vi "ep_Load Torque Efficiency (1 Chan).vi"(1 "additional efficiency information":T1, 7 "speed [RPM]":dbl, 11 "error in (no error)":errorcluster, 12 "nameplate information":T2, 13 "total input active power [W]":dbl) -> (4 "torque [Nm]":dbl, 6 "load [kW]":dbl, 8 "efficiency [%]":dbl, 15 "error out":errorcluster)   [LabVIEW 2014, in "NI_EP_Motor Monitoring.lvlib"]
uses:
  <vilib>/addons/Electrical Power/Motor Monitoring/NI_EP_Motor Monitoring.lvlib
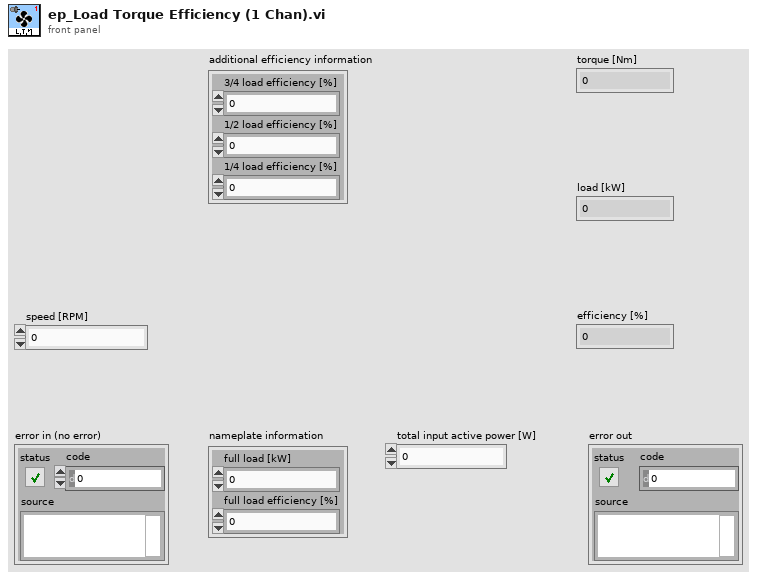
[diagram p1: front panel]
types:
  T1 = cluster{"3/4 load efficiency [%]":dbl, "1/2 load efficiency [%]":dbl, "1/4 load efficiency [%]":dbl}
  T2 = cluster{"full load [kW]":dbl, "full load efficiency [%]":dbl}
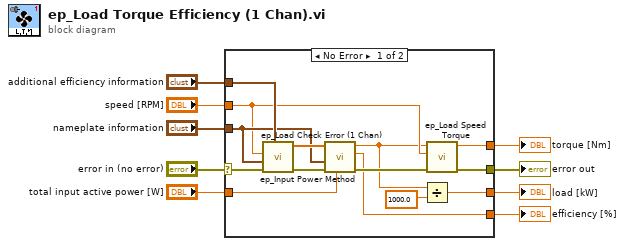
[diagram p0: block diagram]
diagram:
  n1 = case shown="No Error" "error in (no error)" {
    selector: "error in (no error)" -> [w23 w24]
    tunnel: [w15 w24] -> w8
    tunnel: "total input active power [W]" -> [w18 _]
    tunnel: "nameplate information" -> [w19 _]
    tunnel: "speed [RPM]" -> [w16 _]
    tunnel: "additional efficiency information" -> [w22 _]
    tunnel: [w14 _] -> w3
    tunnel: [w11 _] -> w2
    tunnel: [w13 _] -> w1
    frame No Error {
      n2 = call <vilib>:"ep_Load Check Error (1 Chan).vi"("additional efficiency information"=w22, "error in (no error)"=w23, "nameplate information"=w19, "speed [RPM]"=w16) -> ("error out"=w21:errorcluster, "efficiency values [%]"=w20:dbl[])  [unwired: 6 in]
      n3 = call <vilib>:"ep_Input Power Method.vi"("total input active power [W]"=w18, "error in (no error)"=w21, "nameplate information"=w19, "efficiency values [%]"=w20) -> ("error out"=w17:errorcluster, "efficiency [%]"=w13:dbl, "load [W]"=w12:dbl)  [unwired: 5 in]
      n4 = Divide(x=w12, y=1000.0) -> (x/y=w11:dbl)
      n5 = call <vilib>:"ep_Load Speed Torque.vi"("error in (no error)"=w17, "speed [RPM]"=w16, "load [W]"=w12) -> ("error out"=w15:errorcluster, "torque [Nm]"=w14:dbl)  [unwired: 7 in]
    }
    frame Error {
    }
  }
  "error out" <- w8
  "torque [Nm]" <- w3
  "load [kW]" <- w2
  "efficiency [%]" <- w1
